vi "lithographyWorking.vi"() -> ()   [LabVIEW 2016]
uses:
  Controls/lithography_Control.ctl
  litho folder/Global/Lithography Data.vi
panel:
  in  "References":T1
  out "Current Object":string
  out "Status":string
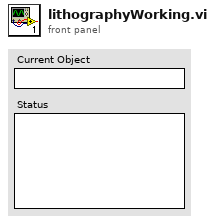
[diagram p1: front panel]
types:
  T1 = cluster{"Scan":refnum<k7>, "Litho":refnum<k7>, "Application":refnum<k7>}
  T2 = cluster{"X_offset":dbl, "Y_offset":dbl, "init_x":dbl, "init_y":dbl, "voltage":dbl}
  T3 = cluster{"Name":string, "Litho":cluster{"X":dbl, "Y":dbl, "Speed":dbl, "Voltage":dbl}[]}[]
  T4 = typedef "lithography_Control.ctl" = enum16{"open_app", "create_ref", "current_pos", "init_litho", "get_init_pt", "clear_litho", "set_param", "move_tip", "create_queue", "clean_up_litho", "start_litho", "end"}
  T5 = cluster{"References":cluster{"Scan":refnum<k7>, "Litho":refnum<k7>, "Application":refnum<k7>}, "Pattern Data":cluster{"Name":string, "Litho":cluster{"X":dbl, "Y":dbl, "Speed":dbl, "Voltage":dbl}[]}, "Values":cluster{"X_offset":dbl, "Y_offset":dbl, "init_x":dbl, "init_y":dbl, "voltage":dbl}}
  T6 = cluster{"X":dbl, "Y":dbl, "Speed":dbl, "Voltage":dbl}[]
  T7 = cluster{"X":dbl, "Y":dbl, "Speed":dbl, "Voltage":dbl}
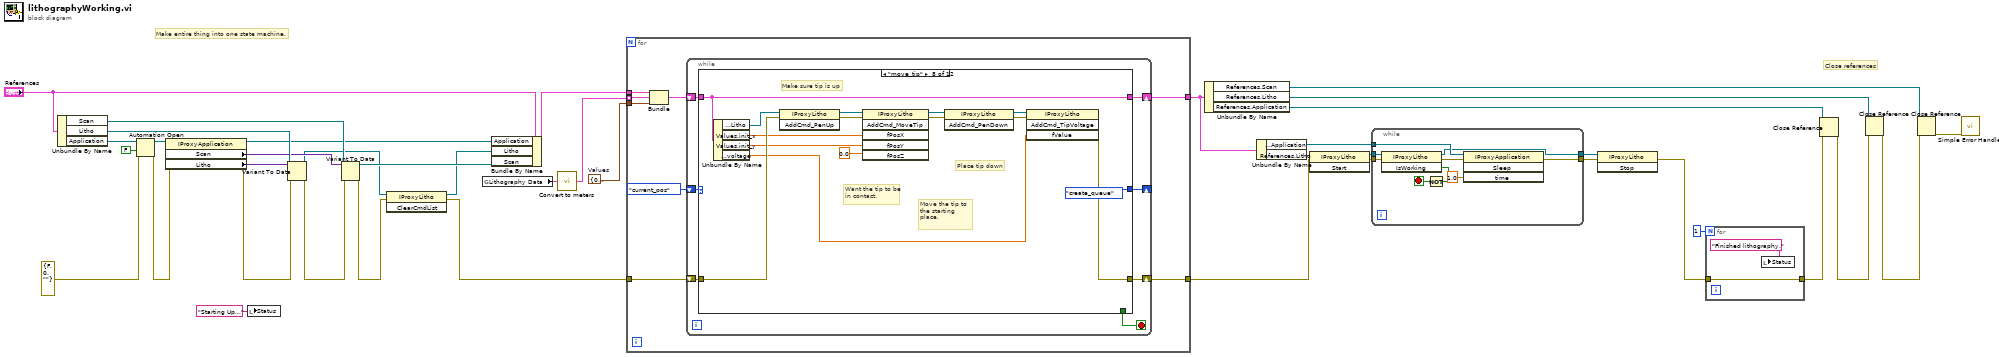
[diagram p0: block diagram]
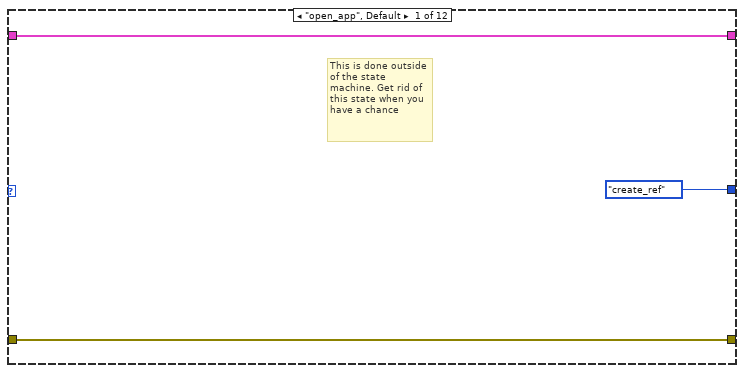
[diagram p2: hidden frame]
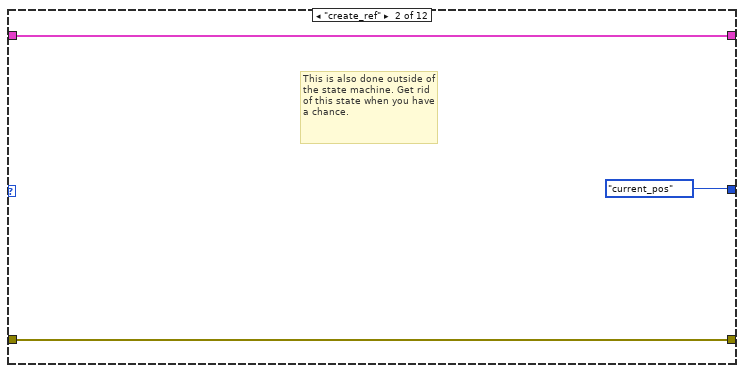
[diagram p3: hidden frame]
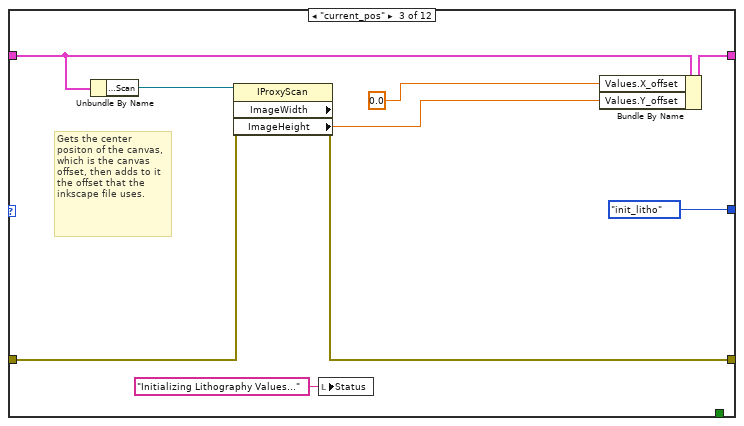
[diagram p4: hidden frame]
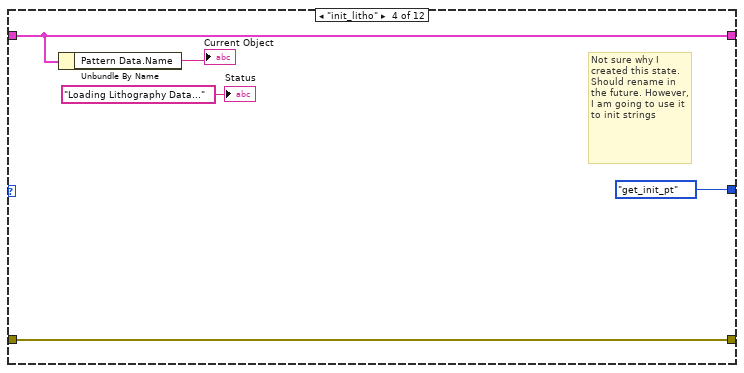
[diagram p5: hidden frame]
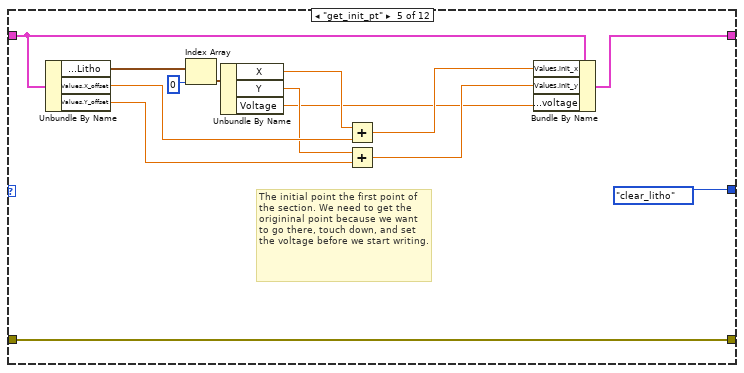
[diagram p6: hidden frame]
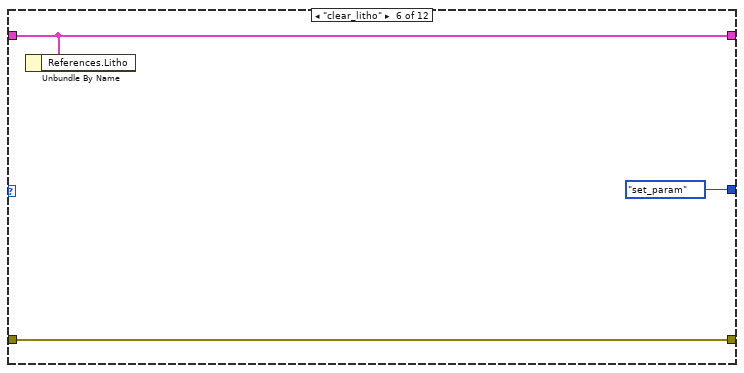
[diagram p7: hidden frame]
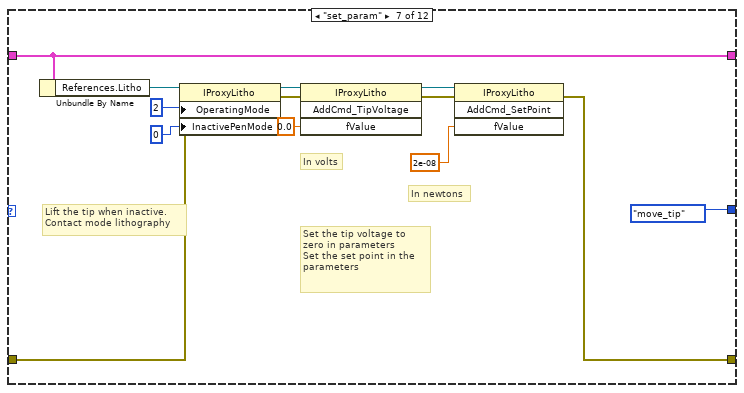
[diagram p8: hidden frame]
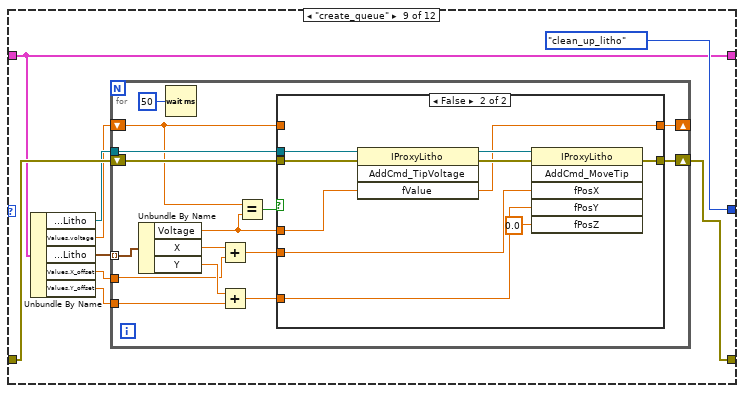
[diagram p9: hidden frame]
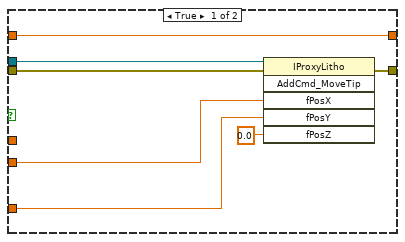
[diagram p10: hidden frame]
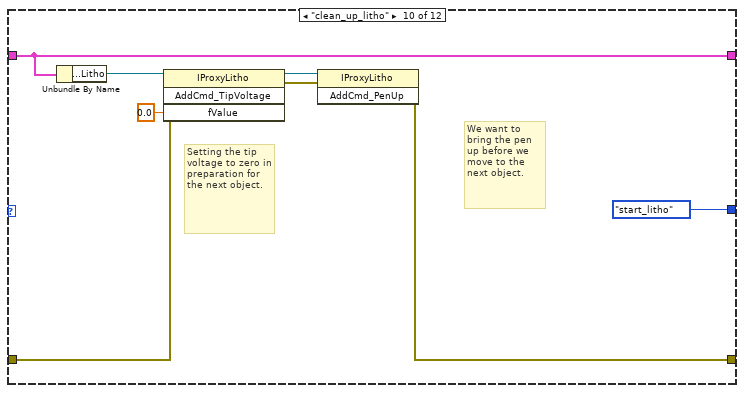
[diagram p11: hidden frame]
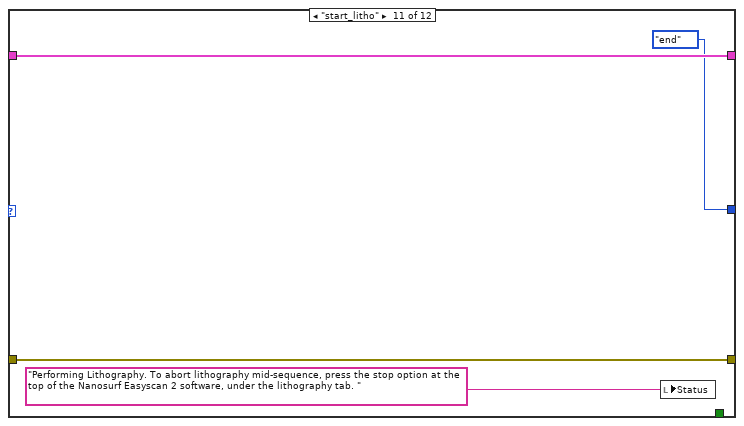
[diagram p12: hidden frame]
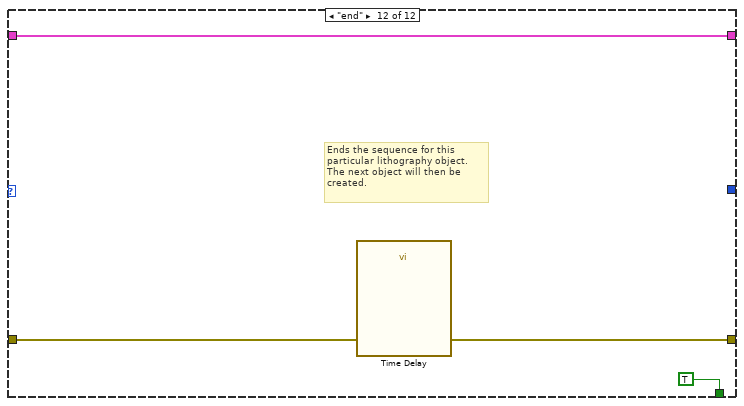
[diagram p13: hidden frame]
diagram:
  w40 = T2 {"X_offset"=0.0, "Y_offset"=0.0, "init_x"=0.0, "init_y"=0.0, "voltage"=0.0}  # Values
  # "Make entire thing into one state machine."
  # "Close references"
  n1 = Unbundle By Name("References") -> ("Scan"=w36:refnum<k7>, "Litho"=w37:refnum<k7>, "Application"=w38:refnum<k7>)
  n2 = Automation Open(error in (no error)=errorcluster {"status"=FALSE, "code"=0, "source"=""}, Automation Refnum=w38, 9:FALSE ("open new instance (false)")) -> (Automation Refnum=w39:refnum<k7>, error out=w24:errorcluster)  [unwired: 1 in]
  n3 = property class="IProxyApplication"(reference=w39, error in=w24) -> (reference out=w35:refnum<k7>, error out=w23:errorcluster, "Scan"=w28:variant, "Litho"=w27:variant)
  n4 = local write "Status"("Starting Up..." ("Status")) -> ()
  n5 = Variant To Data(error in=w23, type=w37, Variant=w27) -> (data=w4:refnum<k7>, error out=w22:errorcluster)
  n6 = Variant To Data(error in=w22, type=w36, Variant=w28) -> (data=w34:refnum<k7>, error out=w2:errorcluster)
  n7 = invoke class="IProxyLitho" method="ClearCmdList"(reference=w4, error in=w2) -> (reference out=w3:refnum<k7>, error out=w1:errorcluster)  [unwired: 1 in, 1 out]
  n8 = global read "Lithography Data.vi" "Lithography Data"() -> (w18:T3)
  n9 = Bundle By Name(cluster="References", "Application"=w35, "Litho"=w3, "Scan"=w34) -> (w33:T1)
  n10 = call "Convert to meters.vi"("Lithography Data In"=w18) -> ("Lithography Data Out"=w14:T3)
  n11 = for {
    tunnel: w33 -> [w46]
    tunnel: w14 -> [w47] mode=indexing
    tunnel: w1 -> [w45]
    tunnel: [w44] -> w5
    tunnel: w40 -> [w43]
    tunnel: [w42] -> w7
    n12 = Bundle("References"=w46, "Pattern Data"=w47, "Values"=w43) -> (w41:T5)  [unwired: 1 in]
    n13 = while {
      shift-right: [w51] -> _
      shift-left: lithography_Control."current_pos" -> [w55]
      shift-right: [w53] -> w42
      shift-left: w41 -> [w54]
      shift-right: [w50] -> w44
      shift-left: w45 -> [w52]
      stop <- w49 stop-if-true
      n14 = case shown="\"move_tip\"" w55 {
        tunnel: w54 -> [w56 w61 w68 w73 w80 w91 w104 w119 w126 w168 w173 w177]
        tunnel: [w56 w61 w67 w73 w79 w91 w104 w119 w126 w168 w173 w177] -> w53
        tunnel: w52 -> [w57 w59 w66 w74 w88 w90 w100 w113 w128 w163 w170 w174]
        tunnel: [lithography_Control."create_ref" lithography_Control."current_pos" lithography_Control."init_litho" lithography_Control."get_init_pt" lithography_Control."clear_litho" lithography_Control."set_param" lithography_Control."move_tip" lithography_Control."create_queue" lithography_Control."clean_up_litho" lithography_Control."start_litho" lithography_Control."end" _] -> w51
        tunnel: [w57 w59 w65 w74 w88 w90 w94 w108 w127 w167 w170 w175] -> w50
        tunnel: [_ _ _ _ _ _ _ _ _ _ _ TRUE] -> w49
        frame "open_app", Default {
          # "This is done outside of the state machine. Get rid of this state when you have a chance"
        }
        frame "create_ref" {
          # "This is also done outside of the state machine. Get rid of this state when you have a chance."
        }
        frame "current_pos" {
          # "Gets the center positon of the canvas, which is the canvas offset, then adds to it the offset that the inkscape file uses."
          n15 = Unbundle By Name(w68) -> ("References.Scan"=w69:refnum<k7>)
          n16 = property class="IProxyScan" props=["ImageWidth", "ImageHeight"](reference=w69, error in=w66) -> (error out=w65:errorcluster, "ImageHeight"=w63:dbl)  [unwired: 2 out]
          n17 = local write "Status"("Initializing Lithography Values..." ("Status")) -> ()
          n18 = Bundle By Name(cluster=w68, "Values.X_offset"=0.0 ("ImageWidth"), "Values.Y_offset"=w63) -> (w67:T5)
        }
        frame "init_litho" {
          # "Not sure why I created this state. Should rename in the future. However, I am going to use it to init strings"
          n19 = Unbundle By Name(w73) -> ("Pattern Data.Name"=→"Current Object":string)
          "Status" <- "Loading Lithography Data..." ("Status")
        }
        frame "get_init_pt" {
          # "The initial point the first point of the section. We need to get the origininal point because we want to go there, touch down, and set the voltage before we start writing."
          n20 = Unbundle By Name(w80) -> ("Pattern Data.Litho"=w86:T6, "Values.X_offset"=w83:dbl, "Values.Y_offset"=w81:dbl)
          n21 = Index Array(array=w86, index=0) -> (element=w85:T7)
          n22 = Unbundle By Name(w85) -> ("X"=w84:dbl, "Y"=w82:dbl, "Voltage"=w76:dbl)
          n23 = Add(x=w84, y=w83) -> (x+y=w78:dbl)
          n24 = Add(x=w82, y=w81) -> (x+y=w77:dbl)
          n25 = Bundle By Name(cluster=w80, "Values.init_x"=w78, "Values.init_y"=w77, "Values.voltage"=w76) -> (w79:T5)
        }
        frame "clear_litho" {
          n26 = Unbundle By Name(w91) -> ()  [unwired: 1 out]
        }
        frame "set_param" {
          # "In volts"
          # "In newtons"
          # "Set the tip voltage to zero in parameters\nSet the set point in the parameters"
          # "Lift the tip when inactive.\nContact mode lithography"
          n27 = Unbundle By Name(w104) -> ("References.Litho"=w103:refnum<k7>)
          n28 = property class="IProxyLitho"(reference=w103, error in=w100, "OperatingMode"=2 ("InactivePenMode"), "InactivePenMode"=0 ("OperatingMode")) -> (reference out=w99:refnum<k7>, error out=w98:errorcluster)
          n29 = invoke class="IProxyLitho" method="AddCmd_TipVoltage"(reference=w99, error in=w98, "fValue"=0.0) -> (reference out=w96:refnum<k7>, error out=w95:errorcluster)  [unwired: 1 in, 2 out]
          n30 = invoke class="IProxyLitho" method="AddCmd_SetPoint"(reference=w96, error in=w95, "fValue"=2e-08 ("SetPoint")) -> (error out=w94:errorcluster)  [unwired: 1 in, 3 out]
        }
        frame "move_tip" {
          # "Want the tip to be in contact."
          # "Make sure tip is up"
          # "Place tip down"
          # "Move the tip to the starting place."
          n31 = Unbundle By Name(w119) -> ("References.Litho"=w112:refnum<k7>, "Values.init_x"=w111:dbl, "Values.init_y"=w110:dbl, "Values.voltage"=w106:dbl)
          n32 = invoke class="IProxyLitho" method="AddCmd_PenUp"(reference=w112, error in=w113) -> (reference out=w118:refnum<k7>, error out=w115:errorcluster)  [unwired: 1 in, 1 out]
          n33 = invoke class="IProxyLitho" method="AddCmd_MoveTip"(reference=w118, error in=w115, "fPosX"=w111, "fPosY"=w110, "fPosZ"=0.0) -> (reference out=w117:refnum<k7>, error out=w114:errorcluster)  [unwired: 1 in, 4 out]
          n34 = invoke class="IProxyLitho" method="AddCmd_PenDown"(reference=w117, error in=w114) -> (reference out=w109:refnum<k7>, error out=w107:errorcluster)  [unwired: 1 in, 1 out]
          n35 = invoke class="IProxyLitho" method="AddCmd_TipVoltage"(reference=w109, error in=w107, "fValue"=w106) -> (error out=w108:errorcluster)  [unwired: 1 in, 3 out]
        }
        frame "create_queue" {
          n36 = Unbundle By Name(w126) -> ("References.Litho"=w122:refnum<k7>, "Values.voltage"=w121:dbl, "Pattern Data.Litho"=w125:T6, "Values.X_offset"=w124:dbl, "Values.Y_offset"=w123:dbl)
          n37 = for {
            shift-right: [w142] -> w127
            shift-left: w128 -> [w143]
            tunnel: w122 -> [w144]
            tunnel: w125 -> [w134] mode=indexing
            tunnel: w124 -> [w135]
            tunnel: w123 -> [w139]
            shift-right: [w131] -> _
            shift-left: w121 -> [w130]
            n38 = Unbundle By Name(w134) -> ("Voltage"=w132:dbl, "X"=w141:dbl, "Y"=w138:dbl)
            n39 = Wait (ms)(milliseconds to wait=u32 50) -> ()  [unwired: 1 out]
            n40 = Add(x=w141, y=w135) -> (x+y=w140:dbl)
            n41 = Add(x=w138, y=w139) -> (x+y=w137:dbl)
            n42 = Equal?(x=w130, y=w132) -> (x = y?=w133:bool)
            n43 = case shown="False" w133 {
              tunnel: w144 -> [w151 w157]
              tunnel: w143 -> [w150 w156]
              tunnel: [w148 w160] -> w142
              tunnel: w140 -> [w147 w159]
              tunnel: w137 -> [w146 w158]
              tunnel: w132 -> [_ w153]
              tunnel: [w145 w152] -> w131
              tunnel: w130 -> [w145 _]
              frame True {
                n44 = invoke class="IProxyLitho" method="AddCmd_MoveTip"(reference=w151, error in=w150, "fPosX"=w147, "fPosY"=w146, "fPosZ"=0.0 ("fPosX")) -> (error out=w148:errorcluster)  [unwired: 1 in, 5 out]
              }
              frame False {
                n45 = invoke class="IProxyLitho" method="AddCmd_TipVoltage"(reference=w157, error in=w156, "fValue"=w153) -> (reference out=w154:refnum<k7>, error out=w155:errorcluster, "fValue"=w152:dbl)  [unwired: 1 in, 1 out]
                n46 = invoke class="IProxyLitho" method="AddCmd_MoveTip"(reference=w154, error in=w155, "fPosX"=w159, "fPosY"=w158, "fPosZ"=0.0 ("fPosX")) -> (error out=w160:errorcluster)  [unwired: 1 in, 5 out]
              }
            }
          }
        }
        frame "clean_up_litho" {
          # "Setting the tip voltage to zero in preparation for the next object."
          # "We want to bring the pen up before we move to the next object."
          n47 = Unbundle By Name(w168) -> ("References.Litho"=w166:refnum<k7>)
          n48 = invoke class="IProxyLitho" method="AddCmd_TipVoltage"(reference=w166, error in=w163, "fValue"=0.0) -> (reference out=w165:refnum<k7>, error out=w164:errorcluster)  [unwired: 1 in, 2 out]
          n49 = invoke class="IProxyLitho" method="AddCmd_PenUp"(reference=w165, error in=w164) -> (error out=w167:errorcluster)  [unwired: 1 in, 2 out]
        }
        frame "start_litho" {
          n50 = local write "Status"("Performing Lithography. To abort lithography mid-sequence, press the stop option at the top of the Nanosurf Easyscan 2 software, under the lithography tab. " ("Status")) -> ()
        }
        frame "end" {
          # "Ends the sequence for this particular lithography object. The next object will then be created."
          n51 = call "Time Delay"("error in (no error)"=w174) -> ("error out"=w175:errorcluster)  [unwired: 10 in]
        }
      }
    }
  }
  n52 = Unbundle By Name(w7) -> ("References.Scan"=w29:refnum<k7>, "References.Litho"=w30:refnum<k7>, "References.Application"=w31:refnum<k7>)
  n53 = Unbundle By Name(w7) -> ("References.Application"=w13:refnum<k7>, "References.Litho"=w8:refnum<k7>)
  n54 = invoke class="IProxyLitho" method="Start"(reference=w8, error in=w5) -> (reference out=w9:refnum<k7>, error out=w10:errorcluster)  [unwired: 1 in, 1 out]
  n55 = while {
    tunnel: w9 -> [w186]
    tunnel: [w178] -> w11
    tunnel: w10 -> [w184]
    tunnel: [w181] -> w12
    tunnel: w13 -> [w180]
    stop <- w183 stop-if-true
    n56 = invoke class="IProxyLitho" method="IsWorking"(reference=w186, error in=w184) -> (reference out=w178:refnum<k7>, error out=w182:errorcluster, "IsWorking"=w185:bool)  [unwired: 1 in]
    n57 = Not(x=w185) -> (.not. x?=w183:bool)
    n58 = invoke class="IProxyApplication" method="Sleep"(reference=w180, error in=w182, "time"=1.0) -> (error out=w181:errorcluster)  [unwired: 1 in, 3 out]
  }
  n59 = invoke class="IProxyLitho" method="Stop"(reference=w11, error in=w12) -> (error out=w6:errorcluster)  [unwired: 1 in, 2 out]
  n60 = for {
    N: 1 -> [_]
    tunnel: w6 -> [w187]
    tunnel: [w187] -> w15
    n61 = local write "Status"("Finished lithography.") -> ()
  }
  n62 = Close Reference(reference=w31, error in (no error)=w15) -> (error out=w21:errorcluster)
  n63 = Close Reference(reference=w30, error in (no error)=w21) -> (error out=w20:errorcluster)
  n64 = Close Reference(reference=w29, error in (no error)=w20) -> (error out=w19:errorcluster)
  n65 = call <vilib>:"Simple Error Handler.vi"("error in (no error)"=w19) -> ()  [unwired: 4 in, 5 out]
